vi "Test_Count.vi"(8 "error in (no error)":errorcluster, 11 "TestCase in":refnum<class "StringList_Delegations.lvclass">) -> (0 "error out":errorcluster, 3 "TestCase out":refnum<class "StringList_Delegations.lvclass">)   [LabVIEW 2009, in "StringList_Delegations.lvclass"]
uses:
  StringList_Delegations.lvclass
  StringList_Delegations.lvclass/StringList_Delegations.ctl
  source/Lists.Interfaces/StringList/StringList.lvclass
  Test Doubles/ListImp_RefSpy/ListImp_RefSpy.lvclass
  UnitTestComparisons/UnitTestComparisons.lvlib
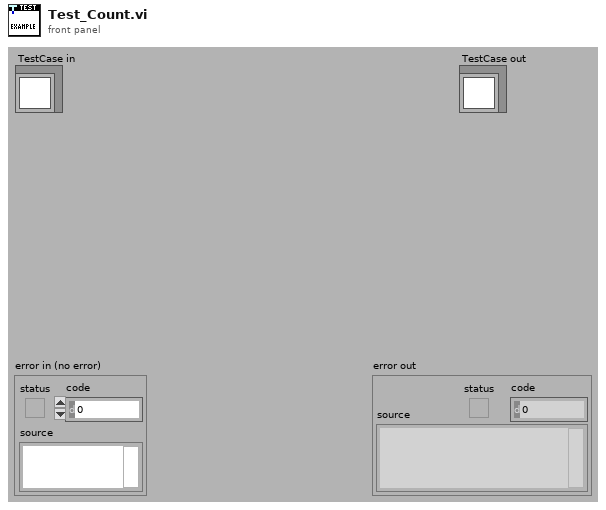
[diagram p1: front panel]
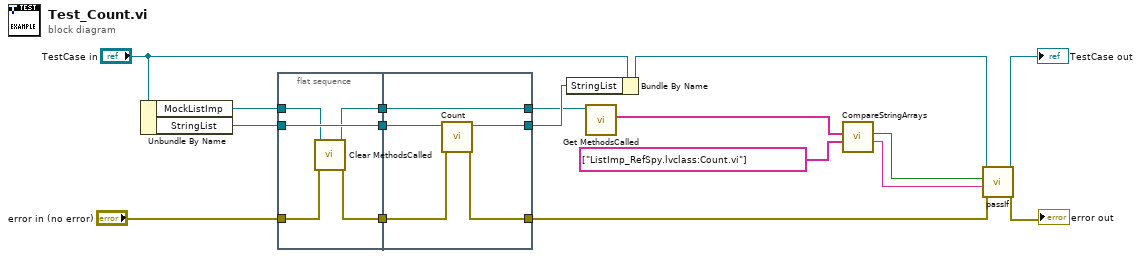
[diagram p0: block diagram]
diagram:
  n1 = Unbundle By Name("TestCase in") -> ("MockListImp"=w12:refnum<class "ListImp_RefSpy.lvclass">, "StringList"=w14:refnum<class "StringList.lvclass">)
  n2 = flat-sequence {
    tunnel: w12 -> [w21]
    tunnel: "error in (no error)" -> [w19]
    tunnel: w14 -> [w22]
    tunnel: [w22] -> w11
    tunnel: [w18] -> w10
    tunnel: [w20] -> w9
    tunnel: w11 -> [w27]
    tunnel: w10 -> [w25]
    tunnel: w9 -> [w23]
    tunnel: [w26] -> w5
    tunnel: [w24] -> w7
    tunnel: [w23] -> w6
    frame #0 {
      n3 = call "Clear MethodsCalled.vi"("error in (no error)"=w19, "MockListImp in"=w21) -> ("error out"=w18:errorcluster, "MockListImp out"=w20:refnum<class "ListImp_RefSpy.lvclass">)  [unwired: 8 in]
    }
    frame #1 {
      n4 = call-dynamic "Count.vi"("error in (no error)"=w25, "StringList in"=w27) -> ("error out"=w26:errorcluster, "StringList out"=w24:refnum<class "StringList.lvclass">)  [unwired: 7 in, 1 out]
    }
  }
  n5 = Bundle By Name(cluster="TestCase in", "StringList"=w7) -> (w8:refnum<class "StringList_Delegations.lvclass">)
  n6 = call "Get MethodsCalled.vi"("MockListImp"=w6) -> ("MethodsCalled"=w4:string[])  [unwired: 9 in, 1 out]
  n7 = call "CompareStringArrays.vi"("Expected Strings"=string[] ["ListImp_RefSpy.lvclass:Count.vi"] ("MethodsCalled"), "Actual Strings"=w4) -> ("Message"=w1:string, "Equal?"=w2:bool)  [unwired: 8 in]
  n8 = call-dynamic "passIf.vi"("error in (no error)"=w5, "message (\"\")"=w1, "pass"=w2, "TestCase in"=w8) -> ("error out"=→"error out":errorcluster, "TestCase out"=→"TestCase out":refnum<class "StringList_Delegations.lvclass">)  [unwired: 6 in]
